vi "Error Query.vi"(8 "error in (no error)":errorcluster, 11 "VISA resource name":refnum<visa-resource-name>) -> (0 "error out":errorcluster, 1 "Error Message":string, 2 "Error Code":i32[](array[numeric]), 3 "VISA resource name out":refnum<visa-resource-name>)   [LabVIEW 2020, in "Agilent 3458.lvlib"]
doc: "Queries the instrument for any errors in the instrument's error queue. It will continue to read errors until all errors have been read from the instrument. Any errors will be returned in the Error Out cluster.\n\nNote:\nThis VI is called automatically by most driver VIs so it is not usually necessary to call this in an application."
uses:
  Agilent 3458.lvlib
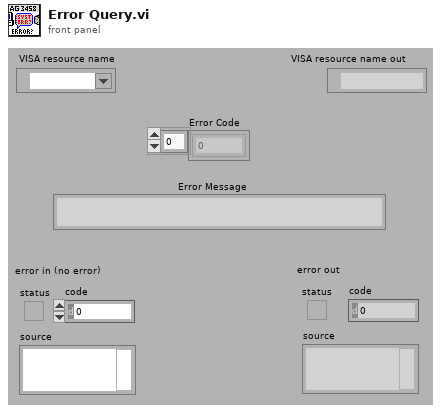
[diagram p1: front panel]
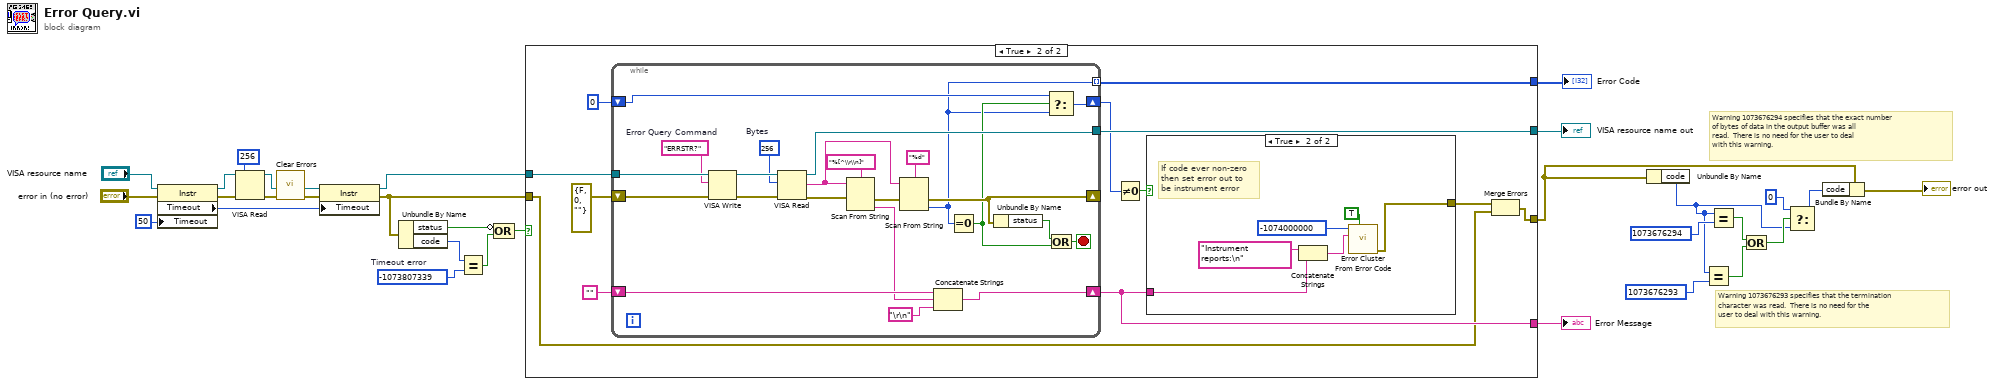
[diagram p0: block diagram]
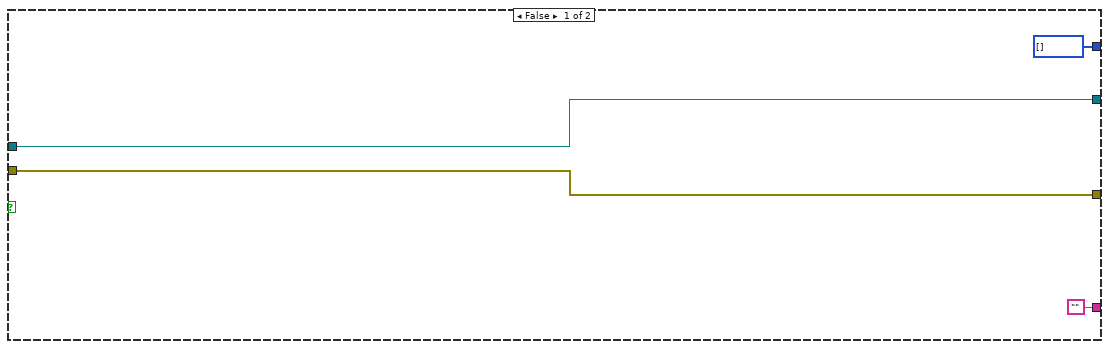
[diagram p2: hidden frame]
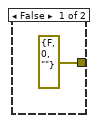
[diagram p3: hidden frame]
diagram:
  w28 = -1073807339  # Timeout error
  # "Warning 1073676293 specifies that the termination \ncharacter was read.  There is no need for the \nuser to deal with this warning."
  # "Warning 1073676294 specifies that the exact number\nof bytes of data in the output buffer was all\nread.  There is no need for the user to deal\nwith this warning."
  n1 = property class="Instr"(reference="VISA resource name", error in="error in (no error)", "Timeout"=u32 50 ("General Settings:Timeout Value")) -> (reference out=w6:refnum<visa-resource-name>, error out=w7:errorcluster, "Timeout"=w3:u32)
  n2 = VISA Read(VISA resource name=w6, byte count=u32 256, error in (no error)=w7) -> (VISA resource name out=w5:refnum<visa-resource-name>, error out=w2:errorcluster)  [unwired: 2 out]
  n3 = call <vilib>:"Clear Errors.vi"("error in (no error)"=w2) -> ("error out"=w1:errorcluster)  [unwired: 5 in, 1 out]
  n4 = property class="Instr"(reference=w5, error in=w1, "Timeout"=w3) -> (reference out=w8:refnum<visa-resource-name>, error out=w10:errorcluster)
  n5 = Unbundle By Name(w10) -> ("status"=w29:bool, "code"=w26:i32)
  n6 = Equal?(x=w26, y=w28) -> (x = y?=w27:bool)
  n7 = Compound Arithmetic op=OR(invert w29, w27) -> (w25:bool)
  n8 = case shown="True" w25 {
    tunnel: [w34 w46] -> w30
    tunnel: w8 -> [w34 w45]
    tunnel: w10 -> [w33 w35]
    tunnel: [w33 w43] -> w14
    tunnel: ["" w37] -> w24
    tunnel: [i32[] [] w36] -> w23
    frame False {
    }
    frame True {
      n9 = while {
        tunnel: [w76] -> w46
        tunnel: w45 -> [w75]
        shift-right: [w63] -> w37
        shift-left: "" -> [w66]
        shift-right: [w61] -> w38
        shift-left: 0 -> [w62]
        shift-right: [w59] -> _
        shift-left: errorcluster {"status"=FALSE, "code"=0, "source"=""} ("error in (no error)") -> [w60]
        tunnel: [w54] -> w36 mode=indexing
        stop <- w69 stop-if-true
        w73 = u32 256  # Bytes
        w71 = "ERRSTR?"  # Error Query Command
        n10 = VISA Write(VISA resource name=w75, write buffer=w71, error in (no error)=w60) -> (VISA resource name out=w74:refnum<visa-resource-name>, error out=w72:errorcluster)  [unwired: 1 out]
        n11 = VISA Read(VISA resource name=w74, byte count=w73, error in (no error)=w72) -> (VISA resource name out=w76:refnum<visa-resource-name>, read buffer=w67:string, error out=w58:errorcluster)  [unwired: 1 out]
        n12 = Scan From String(format string="%[^\\r\\n]", input string=w67, error in=w58) -> (error out=w57:errorcluster, output 1=w64:string)  [unwired: 2 in, 2 out]
        n13 = Scan From String(format string="%d", input string=w67, error in=w57) -> (error out=w59:errorcluster, output 1=w54:i32)  [unwired: 2 in, 2 out]
        n14 = Concatenate Strings(w66, w64, "\r\n") -> (w63:string)
        n15 = Equal To 0?(x=w54) -> (x = 0?=w55:bool)
        n16 = Unbundle By Name(w59) -> ("status"=w56:bool)
        n17 = Select(t=w62, s=w55, f=w54) -> (s? t:f=w61:i32)
        n18 = Or(x=w56, y=w55) -> (x .or. y?=w69:bool)
      }
      n19 = Not Equal To 0?(x=w38) -> (x != 0?=w41:bool)
      n20 = case shown="True" w41 {
        tunnel: w37 -> [_ w52]
        tunnel: [errorcluster {"status"=FALSE, "code"=0, "source"=""} ("error out") w48] -> w40
        frame False {
        }
        frame True {
          # "If code ever non-zero\nthen set error out to\nbe instrument error"
          n21 = Concatenate Strings("Instrument reports:\n" ("Source"), w52) -> (w49:string)
          n22 = call <vilib>:"Error Cluster From Error Code.vi"("show call chain? (False)"=TRUE, "error message (\"\")"=w49, "error code (0)"=-1074000000 ("Code")) -> ("error out"=w48:errorcluster)  [unwired: 6 in]
        }
      }
      n23 = Merge Errors(w40, w35) -> (w43:errorcluster)
    }
  }
  "VISA resource name out" <- w30
  "Error Message" <- w24
  "Error Code" <- w23
  n24 = Unbundle By Name(w14) -> ("code"=w15:i32)
  n25 = Equal?(x=w15, y=1073676293) -> (x = y?=w18:bool)
  n26 = Equal?(x=w15, y=1073676294) -> (x = y?=w17:bool)
  n27 = Or(x=w17, y=w18) -> (x .or. y?=w16:bool)
  n28 = Select(t=0, s=w16, f=w15) -> (s? t:f=w20:i32)
  n29 = Bundle By Name(cluster=w14, "code"=w20) -> (→"error out":errorcluster)
